vi "Custom Icon Editor path token name--Constant.vi"() -> (3 "Custom Icon Editor path token name":string)   [LabVIEW 2021]
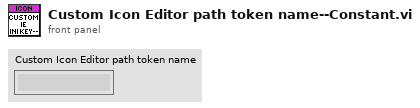
[diagram p1: front panel]
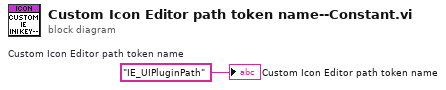
[diagram p0: block diagram]
diagram:
  w1 = "IE_UIPluginPath"  # Custom Icon Editor path token name
  "Custom Icon Editor path token name" <- w1
